vi "settle-detect.vi"(6 "error-max":sgl format="%#_13g", 7 "reset":bool, 8 "settled-samples\nthreshold":u16, 11 "err(k)":sgl) -> (0 "has-settled":bool, 3 "number-settled-samples":u16)   [LabVIEW 2017]
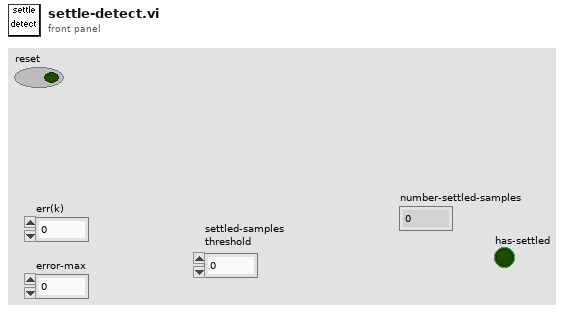
[diagram p1: front panel]
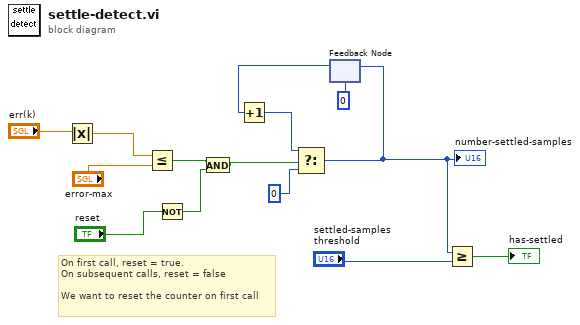
[diagram p0: block diagram]
diagram:
  # "On first call, reset = true.\nOn subsequent calls, reset = false\n\nWe want to reset the counter on first call"
  n1 = Absolute Value(x="err(k)") -> (abs(x)=w6:sgl)
  n2 = Less Or Equal?(x=w6, y="error-max") -> (x <= y?=w3:bool)
  n3 = Not(x="reset") -> (.not. x?=w2:bool)
  n4 = And(x=w3, y=w2) -> (x .and. y?=w4:bool)
  n5 = feedback #1(u16 0 ("f")) -> (w13:u16)
  n6 = Increment(x=w13) -> (x+1=w11:u16)
  n7 = Select(t=w11, s=w4, f=u16 0) -> (s? t:f=w9:u16)
  "number-settled-samples" <- w9
  n8 = feedback-in #1(w9) -> ()
  n9 = Greater Or Equal?(x=w9, y="settled-samples\nthreshold") -> (x >= y?=→"has-settled":bool)
